vi "Stop.vi"() -> ()   [LabVIEW 2011]
panel:
  in  "stop":bool
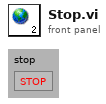
[diagram p1: front panel]
diagram:
